vi "MPB comm protocol.vi"() -> ()   [LabVIEW 2020]
uses:
  controls/comm protocol auto ethernet.ctl
panel:
  out "value":T1={"MPB IP Address"="192.168.1.9", "MPB VLAN"="1", "MPB Port"="11111", "PCP IP Address"="192.168.1.123", "PC VLAN"="1", "PC Port"="11112"}
  in  "Communication Protocol Automotive Ethernet":T1
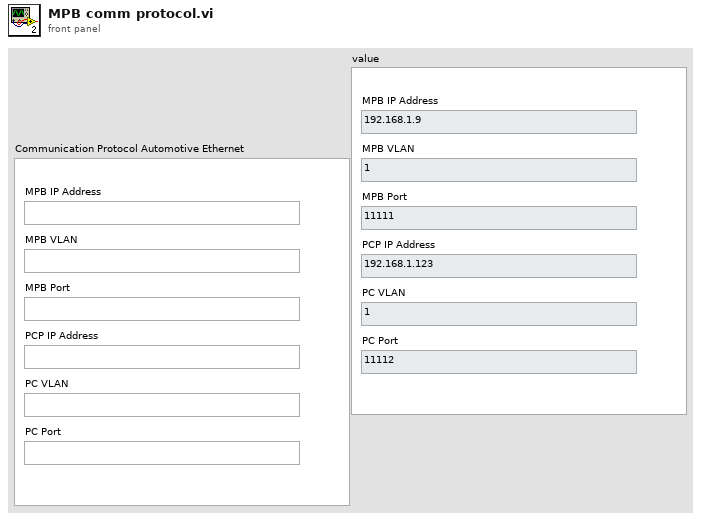
[diagram p1: front panel]
types:
  T1 = typedef "comm protocol auto ethernet.ctl" = cluster{"MPB IP Address":string, "MPB VLAN":string, "MPB Port":string, "PCP IP Address":string, "PC VLAN":string, "PC Port":string}
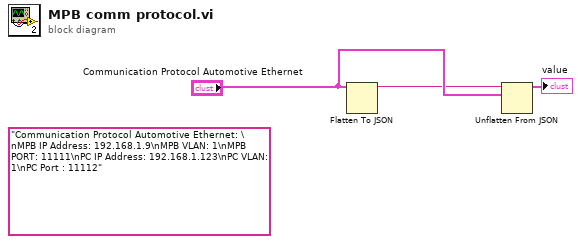
[diagram p0: block diagram]
diagram:
  (unwired) "Communication Protocol Automotive Ethernet: \nMPB IP Address: 192.168.1.9\nMPB VLAN: 1\nMPB PORT: 11111\nPC IP Address: 192.168.1.123\nPC VLAN: 1\nPC Port : 11112"
  n1 = Flatten To JSON(anything="Communication Protocol Automotive Ethernet") -> (JSON string=w2:string)  [unwired: 2 in, 1 out]
  n2 = Unflatten From JSON(JSON string=w2, type and defaults="Communication Protocol Automotive Ethernet") -> (value=→"value":T1)  [unwired: 5 in, 1 out]
